vi "DAQ.vi"() -> ()   [LabVIEW 2024]
uses:
  <vilib>/Instr/_visa.llb/VISA Configure Serial Port (Instr).vi
panel:
  in  "Wave Type":T1(ring)
  in  "Frequency":dbl(slide) scale=1.0..100.0
  out "Write String":string
  out "Waveform Chart":dbl(graph)
  out "Read String":string
  in  "VISA resource":refnum<visa-resource-name>
  in  "stop":bool
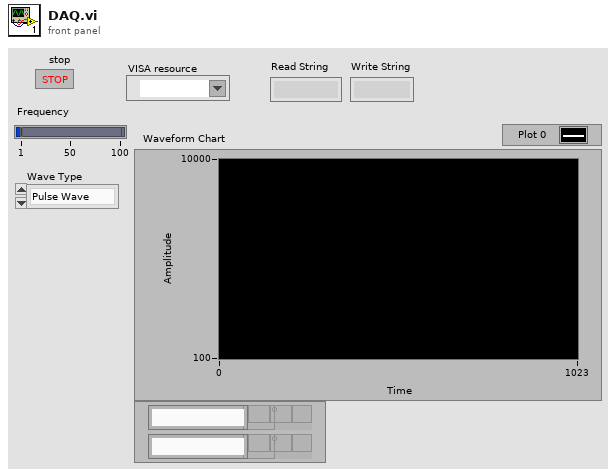
[diagram p1: front panel]
types:
  T1 = enum16{"Pulse Wave", "Consine Wave", "Triangle Wave", "Saw Wave"}
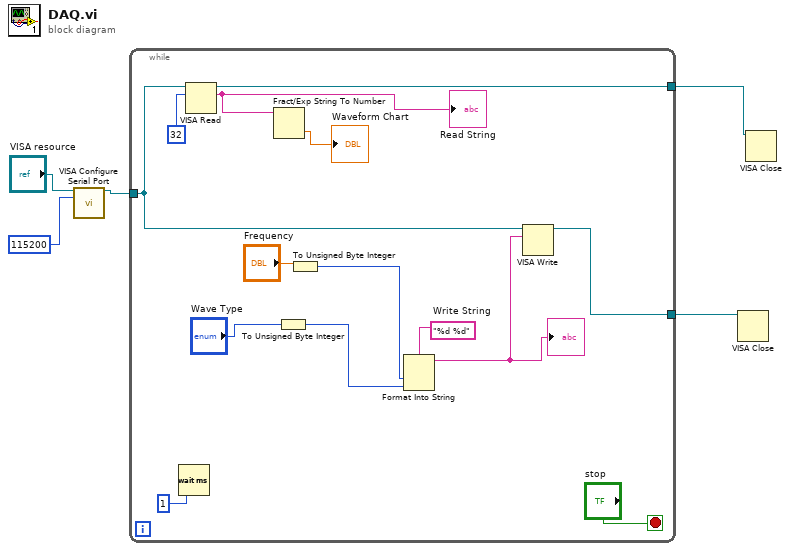
[diagram p0: block diagram]
diagram:
  n1 = call-poly "VISA Configure Serial Port"("VISA resource name"="VISA resource", "baud rate (9600)"=u32 115200) -> ("VISA resource name out"=w2:refnum<visa-resource-name>)  [unwired: 12 in, 1 out]
  n2 = while {
    tunnel: w2 -> [w6]
    tunnel: [w17] -> w3
    tunnel: [w7] -> w1
    stop <- "stop" stop-if-true
    n3 = Wait (ms)(milliseconds to wait=u32 1) -> ()  [unwired: 1 out]
    n4 = VISA Read(VISA resource name=w6, byte count=u32 32) -> (VISA resource name out=w17:refnum<visa-resource-name>, read buffer=w15:string)  [unwired: 1 in, 2 out]
    "Read String" <- w15
    n5 = Fract/Exp String To Number(string=w15) -> (number=→"Waveform Chart":dbl)  [unwired: 3 in, 1 out]
    n6 = To Unsigned Byte Integer(number="Wave Type") -> (unsigned 8bit integer=w9:u8)
    n7 = To Unsigned Byte Integer(number="Frequency") -> (unsigned 8bit integer=w10:u8)
    n8 = Format Into String(format string="%d %d", w10, w9) -> (resulting string=w8:string)  [unwired: 2 in, 1 out]
    "Write String" <- w8
    n9 = VISA Write(VISA resource name=w6, write buffer=w8) -> (VISA resource name out=w7:refnum<visa-resource-name>)  [unwired: 1 in, 2 out]
  }
  n10 = VISA Close(VISA resource name=w1) -> ()  [unwired: 1 in, 1 out]
  n11 = VISA Close(VISA resource name=w3) -> ()  [unwired: 1 in, 1 out]
